vi "RLC Circuit.vi"() -> ()   [LabVIEW 2017]
uses:
  <vilib>/addons/_JKI.lib/REST Client/classes/REST Client/HTTP Header.ctl
  <vilib>/addons/_JKI.lib/REST Client/classes/REST Client/REST Client.lvclass
  <vilib>/httpClient/MultipartData.ctl
  <vilib>/LVH/i3 JSON/JSON Parsing/Get Object Parameter Files/Get Object Parameter - Object.vi
  <vilib>/LVH/i3 JSON/JSON Generation/Create Value Files/Create Value - String.vi
  <vilib>/LVH/i3 JSON/JSON Generation/Add Object Parameter Files/Add Object Parameter - Object.vi
  <vilib>/Analysis/NI_AALBase.lvlib
  <vilib>/httpClient/LabVIEWHTTPClient.lvlib
  <vilib>/LVH/i3 JSON/i3-json.lvlib
panel:
  out "error out  2":errorcluster
  out "Local Cluster":T2={"Base URL Getting"="https://api.dev.enlil.io/api", "Path"="/v1/document_revisions/external/ALI00017/draft", "Default Headers ([JSON])"=[{"header"="Content-Type", "value"="application/json"}, {"header"="Authorization", "value"="apitoken 2096a662-4947-42f5-97bc-84cfdf20fe4e:bc240510-8f48-43e3-889a-471659905c2e"}]}
  out "error out 4":errorcluster={"status"=TRUE, "code"=0, "source"="Input has UNKNOWN type, Expecting JSON Object"}
  out "headers":string="HTTP/1.1 201 Created\r\nDate: Wed, 04 Mar 2020 22:35:49 GMT\r\nContent-Type: application/json; charset=utf-8\r\nContent-Length: 655\r\nConnection: keep-alive\r\nSet-Cookie: AWSALB=VxqNwSYeQG0m47IXiOZ1OzDZLcK+M/95m4sL+aiBIfyiuOveEpJhbIw2+MdgPGt87DC4Ig6JZd2B6jRkdLsrHcqbrtdnjQCVFvEQhCU/fEw1chZBYJ72zQdVEr3j; Expires=Wed, 11 Mar 2020 22:35:48 GMT; Path=/\r\nSet-Cookie: AWSALBCORS=VxqNwSYeQG0m47IXiOZ1OzDZLcK+M/95m4sL+aiBIfyiuOveEpJhbIw2+MdgPGt87DC4Ig6JZd2B6jRkdLsrHcqbrtdnjQCVFvEQhCU/fEw1chZBYJ72zQdVEr3j; Expires=Wed, 11 Mar 2020 22:35:48 GMT; Path=/; SameSite=None; Secure\r\nX-Powered-By: Express\r\nAccess-Control-Allow-Origin: *\r\nStrict-Transport-Security: max-age=15552000; includeSubDomains\r\nETag: W/\"28f-tuCZSSTEEmLl4gD3j85fY8Z3L9M\"\r\nVary: Accept-Encoding\r\n\r\n"
  out "error out 3":errorcluster
  in  "Tab Control":enum32{"Page 1", "Page 2"}(tab)
  in  "Start Sending":bool
  in  "Default Headers ([JSON])":T1[](array[typedef])=[{"header"="Content-Type", "value"="application/json"}, {"header"="Authorization", "value"="apitoken 2096a662-4947-42f5-97bc-84cfdf20fe4e:bc240510-8f48-43e3-889a-471659905c2e"}]
  in  "Base URL Getting":string="https://api.dev.enlil.io/api"
  in  "Path":string="/v1/document_revisions/external/ALI00017/draft"
  in  "Start Getting":bool
  out "Status Code":u16=200
  out "Status String":string="OK\r"
  in  "input cluster":T3={"Parameter Name Vin"="vin-k7ad0tyd", "Parameter Name R"="r-k7ad0z99", "Parameter Name L"="l-k7ad13xp", "Parameter Name C"="c-k7ad19ix"}
  in  "Parameter Name All":string="formInput"
  out "Vin":dbl
  out "R":dbl
  out "L":dbl
  out "C":dbl
  out "Response body":string="{\"createdAt\":\"2020-03-02T11:12:30.271Z\",\"updatedAt\":\"2020-03-04T22:15:54.912Z\",\"id\":\"483b4210-fea0-4e5f-86e6-7e2e9ef14ab9\",\"version\":1,\"revision\":1,\"revisionStage\":1,\"description\":\"<p>Luka - RLC _ TEST</p>\",\"name\":\"Luka\",\"status\":\"DRAFT\",\"deprecatedAt\":null,\"releasedAt\":null,\"obsoletedAt\":null,\"retrain\":false,\"formInput\":{\"vin-k7ad0tyd\":\"25\",\"r-k7ad0z99\":\"50\",\"l-k7ad13xp\":\"30\",\"c-k7ad19ix\":\"15\"},\"revisionChangeType\":\"NEXT_REVISION\",\"externalId\":null,\"renderHTML\":null,\"owner\":{\"createdAt\":\"2020-02-19T17:50:40.752Z\",\"updatedAt\":\"2020-02-19T17:50:40.752Z\",\"id\":\"796961dc-c686-4253-97f2-59d9360d9127\",\"active\":true,\"slackUserId\":null,\"user\":{\"createdAt\":\"2020-02-19T17:50:40.752Z\",\"updatedAt\":\"2020-02-19T17:50:40.752Z\",\"id\":\"70b289fa-7831-4846-97f9-a0727380590c\",\"email\":\"luka.stosic+labview@codecons.com\",\"name\":\"Company Admin\",\"permissions\":null,\"avatar\":null}},\"document\":{\"createdAt\":\"2020-03-02T11:12:30.271Z\",\"updatedAt\":\"2020-03-02T11:12:30.271Z\",\"id\":\"7317e6be-3b89-4428-84bb-8531eddc6023\",\"docId\":\"ALI00017\",\"documentType\":{\"createdAt\":\"2020-03-02T09:53:29.165Z\",\"updatedAt\":\"2020-03-02T09:53:29.165Z\",\"id\":\"f5ab57be-8a87-4427-8a37-ad589c6c9a93\",\"documentTypeName\":\"Ali Document\",\"documentTypeAcronym\":\"ALI\",\"group\":\"OTHER\",\"privateNumberPool\":false,\"isQms\":true,\"startingNumber\":1,\"pageDetails\":null},\"referencedBy\":[],\"securityEmployees\":[],\"securityGroups\":[{\"createdAt\":\"2020-02-19T17:50:40.752Z\",\"updatedAt\":\"2020-03-02T11:11:52.054Z\",\"id\":\"e9b1c157-b17b-42e6-940a-b3ff64f3c84a\",\"name\":\"Everyone\",\"permissions\":[\"EMPLOYEE_GET\"],\"defaultForNewUsers\":true,\"tags\":[\"QMS_DEFAULT\",\"OWNERSHIP_CHANGE\"],\"isOfficial\":true,\"employees\":[{\"createdAt\":\"2020-02-19T18:14:19.813Z\",\"updatedAt\":\"2020-02-19T18:14:19.813Z\",\"id\":\"14618d18-3c6c-4a3d-854c-2505bd3d66b8\",\"active\":true,\"slackUserId\":null,\"user\":{\"createdAt\":\"2019-12-17T16:55:55.030Z\",\"updatedAt\":\"2019-12-17T16:55:58.645Z\",\"id\":\"ccba97cc-6396-4955-b83a-8af76ff01aa4\",\"email\":\"adarkazanli@shifamed.com\",\"name\":\"Ammar Darkazanli - Admin\",\"permissions\":null,\"avatar\":null}},{\"createdAt\":\"2020-02-19T17:50:40.752Z\",\"updatedAt\":\"2020-02-19T17:50:40.752Z\",\"id\":\"796961dc-c686-4253-97f2-59d9360d9127\",\"active\":true,\"slackUserId\":null,\"user\":{\"createdAt\":\"2020-02-19T17:50:40.752Z\",\"updatedAt\":\"2020-02-19T17:50:40.752Z\",\"id\":\"70b289fa-7831-4846-97f9-a0727380590c\",\"email\":\"luka.stosic+labview@codecons.com\",\"name\":\"Company Admin\",\"permissions\":null,\"avatar\":null}}]}],\"canAccess\":true},\"referenceTo\":[],\"changeRequest\":null,\"trainingRecords\":[],\"pdf\":null,\"attachments\":[],\"formTemplate\":null,\"formDocument\":{\"createdAt\":\"2020-03-02T11:11:42.254Z\",\"updatedAt\":\"2020-03-02T11:11:52.054Z\",\"id\":\"59fcbba9-0bd2-42e5-afd8-1e80379511c7\",\"version\":1,\"revision\":1,\"revisionStage\":1,\"description\":\"<p><span style=\\\"color: rgb(77,77,77);background-color: rgb(255,255,255);font-size: 14px;font-family: Open Sans\\\", sans-serif;\\\">RLC circuit which imports the data from the api ( Vin - R - L - C ) and exports 2 images to the api. One for Series Circuit and another for Parallel Circuit.</span></p>\",\"name\":\"RLC - Luka Test\",\"status\":\"RELEASED\",\"deprecatedAt\":null,\"releasedAt\":\"2020-03-02T11:11:53.929Z\",\"obsoletedAt\":null,\"retrain\":false,\"formInput\":null,\"revisionChangeType\":\"NEXT_REVISION\",\"externalId\":null,\"renderHTML\":null,\"formTemplate\":{\"createdAt\":\"2020-03-02T11:11:42.254Z\",\"updatedAt\":\"2020-03-02T11:11:42.254Z\",\"id\":\"64323185-9de3-4394-af92-7432be18ca58\",\"schema\":[{\"type\":\"textfield\",\"index\":0,\"name\":\"vin-k7ad0tyd\",\"label\":\"Vin\",\"rules\":\"\",\"applicableOn\":[\"ON_STATE_TO_IN_REVIEW\"],\"formValuesRules\":{}},{\"type\":\"textfield\",\"index\":1,\"name\":\"r-k7ad0z99\",\"label\":\"R\",\"rules\":\"\",\"applicableOn\":[\"ON_STATE_TO_IN_REVIEW\"],\"formValuesRules\":{}},{\"type\":\"textfield\",\"index\":2,\"name\":\"l-k7ad13xp\",\"label\":\"L\",\"rules\":\"\",\"applicableOn\":[\"ON_STATE_TO_IN_REVIEW\"],\"formValuesRules\":{}},{\"type\":\"textfield\",\"index\":3,\"name\":\"c-k7ad19ix\",\"label\":\"C\",\"rules\":\"\",\"applicableOn\":[\"ON_STATE_TO_IN_REVIEW\"],\"formValuesRules\":{}}]},\"document\":{\"createdAt\":\"2020-03-02T11:11:42.254Z\",\"updatedAt\":\"2020-03-02T11:11:42.254Z\",\"id\":\"307b5404-5fb5-4901-b94d-3c29afee9a02\",\"docId\":\"FM00016\"}}}"
  out "error out":errorcluster
  in  "PUT Path":string="/v1/document_revisions/external/0b9ed9ad-4393-4a37-838e-578edaaebe9e"
  out "Response body Putting":string="{\"createdAt\":\"2020-02-22T11:56:35.610Z\",\"updatedAt\":\"2020-03-04T22:35:50.355Z\",\"id\":\"0b9ed9ad-4393-4a37-838e-578edaaebe9e\",\"version\":1,\"revision\":1,\"revisionStage\":1,\"description\":\"<p>Test Ali</p>\",\"name\":\"Test Ali\",\"status\":\"DRAFT\",\"deprecatedAt\":null,\"releasedAt\":null,\"obsoletedAt\":null,\"retrain\":false,\"formInput\":{\"r-1-k6tm7v7p\":\"300,000000\",\"r-2-k6tm82gj\":\"220,000000\",\"r-3-k6tm86pp\":\"700,000000\",\"r-4-k6tm8czn\":\"1200,000000\",\"vin-k6tm7pik\":\"110,000000\",\"vout-k6tm8iia\":\"-22,935223\"},\"revisionChangeType\":\"NEXT_REVISION\",\"externalId\":null,\"renderHTML\":null,\"owner\":{\"createdAt\":\"2020-02-19T17:50:40.752Z\",\"updatedAt\":\"2020-02-19T17:50:40.752Z\",\"id\":\"796961dc-c686-4253-97f2-59d9360d9127\",\"active\":true,\"slackUserId\":null,\"user\":{\"createdAt\":\"2020-02-19T17:50:40.752Z\",\"updatedAt\":\"2020-02-19T17:50:40.752Z\",\"id\":\"70b289fa-7831-4846-97f9-a0727380590c\",\"email\":\"luka.stosic+labview@codecons.com\",\"name\":\"Company Admin\",\"permissions\":null,\"avatar\":null}},\"document\":{\"createdAt\":\"2020-02-22T11:56:35.610Z\",\"updatedAt\":\"2020-02-22T11:56:35.610Z\",\"id\":\"575eb1d7-b8d2-41b8-9d9e-9423dadb7d63\",\"docId\":\"CP00004\",\"documentType\":{\"createdAt\":\"2020-02-19T17:50:40.752Z\",\"updatedAt\":\"2020-02-19T17:50:40.752Z\",\"id\":\"baa29555-e386-488c-b5c3-d6ee972e153c\",\"documentTypeName\":\"Clinical Protocol\",\"documentTypeAcronym\":\"CP\",\"group\":\"OTHER\",\"privateNumberPool\":false,\"isQms\":true,\"startingNumber\":1,\"pageDetails\":null},\"referencedBy\":[],\"securityEmployees\":[],\"securityGroups\":[],\"canAccess\":true},\"referenceTo\":[],\"changeRequest\":null,\"trainingRecords\":[],\"pdf\":null,\"attachments\":[],\"formTemplate\":null,\"formDocument\":{\"createdAt\":\"2020-02-20T20:27:52.637Z\",\"updatedAt\":\"2020-02-24T13:01:24.572Z\",\"id\":\"75c93c40-92be-411d-bc74-84a119fc04b8\",\"version\":2,\"revision\":2,\"revisionStage\":1,\"description\":\"<p>test</p>\",\"name\":\"Form Notebook\",\"status\":\"DEPRECATED\",\"deprecatedAt\":\"2020-02-24T13:01:25.722Z\",\"releasedAt\":\"2020-02-20T20:28:22.146Z\",\"obsoletedAt\":null,\"retrain\":false,\"formInput\":null,\"revisionChangeType\":\"NEXT_REVISION\",\"externalId\":null,\"renderHTML\":null,\"formTemplate\":{\"createdAt\":\"2020-02-20T20:27:52.637Z\",\"updatedAt\":\"2020-02-20T20:27:52.637Z\",\"id\":\"9a42de21-a365-4d40-b1db-612758cdd974\",\"schema\":[{\"type\":\"textfield\",\"index\":0,\"name\":\"vin-k6tm7pik\",\"label\":\"Vin\",\"rules\":\"\",\"applicableOn\":[\"ON_STATE_TO_IN_REVIEW\"],\"formValuesRules\":{}},{\"type\":\"textfield\",\"index\":1,\"name\":\"r-1-k6tm7v7p\",\"label\":\"R1\",\"rules\":\"\",\"applicableOn\":[\"ON_STATE_TO_IN_REVIEW\"],\"formValuesRules\":{}},{\"type\":\"textfield\",\"index\":2,\"name\":\"r-2-k6tm82gj\",\"label\":\"R2\",\"rules\":\"\",\"applicableOn\":[\"ON_STATE_TO_IN_REVIEW\"],\"formValuesRules\":{}},{\"type\":\"textfield\",\"index\":3,\"name\":\"r-3-k6tm86pp\",\"label\":\"R3\",\"rules\":\"\",\"applicableOn\":[\"ON_STATE_TO_IN_REVIEW\"],\"formValuesRules\":{}},{\"type\":\"textfield\",\"index\":4,\"name\":\"r-4-k6tm8czn\",\"placeholder\":\"\",\"label\":\"R4\",\"rules\":\"\",\"applicableOn\":[\"ON_STATE_TO_IN_REVIEW\"],\"formValuesRules\":{}},{\"type\":\"textfield\",\"index\":5,\"name\":\"vout-k6tm8iia\",\"label\":\"Vout\",\"rules\":\"\",\"applicableOn\":[\"ON_STATE_TO_IN_REVIEW\"],\"formValuesRules\":{}},{\"type\":\"textfield\",\"index\":6,\"name\":\"initial-frequency-k6v75gp5\",\"label\":\"Initial Frequency\",\"rules\":\"\",\"applicableOn\":[\"ON_STATE_TO_IN_REVIEW\"],\"formValuesRules\":{}},{\"type\":\"textfield\",\"index\":7,\"name\":\"final-frequency-k6v7609o\",\"label\":\"Final Frequency\",\"rules\":\"\",\"applicableOn\":[\"ON_STATE_TO_IN_REVIEW\"],\"formValuesRules\":{}}]},\"document\":{\"createdAt\":\"2020-02-19T17:54:13.053Z\",\"updatedAt\":\"2020-02-19T17:54:13.053Z\",\"id\":\"316835f7-c3f4-4050-a09b-2d99776d6260\",\"docId\":\"FM00001\"}}}"
  out "Status String":string="OK\r"
  in  "Default Headers ([JSON]) PUT":T1[](array[typedef])=[{"header"="Content-Type", "value"="application/json"}, {"header"="Authorization", "value"="apitoken 2096a662-4947-42f5-97bc-84cfdf20fe4e:bc240510-8f48-43e3-889a-471659905c2e"}]
  in  "Base URL Posting":string="https://api.dev.enlil.io/api"
  in  "Same Params?":bool
  out "Status Code 2":u16=200
  out "body":string="{\"company\":{\"_addresses\":[],\"_acctCodes\":[],\"createdAt\":\"2020-02-19T17:50:40.752Z\",\"updatedAt\":\"2020-02-19T17:50:40.752Z\",\"id\":\"a64ce667-962d-4ce0-9671-2a28305a948e\",\"name\":\"LabView\",\"slackIntegrationEnabled\":true,\"teamId\":null,\"botToken\":null,\"maxRevisionStages\":3,\"numOfDocDigits\":5,\"whiteLabeling\":null,\"remoteValidatorBundleName\":null},\"name\":\"Series\",\"type\":\"png\",\"s3link\":\"a64ce667-962d-4ce0-9671-2a28305a948e/2020-03-04T22:35:49.127Z_Series.png\",\"importMetadataJson\":{},\"cleanCopyStatus\":\"NOT_REQUIRED\",\"s3linkCleanCopy\":null,\"createdAt\":\"2020-03-04T22:35:49.127Z\",\"updatedAt\":\"2020-03-04T22:35:49.127Z\",\"id\":\"7de0ce76-9aaf-4a44-b9a1-fc2d4d2266e7\"}"
  out "ID":string="7de0ce76-9aaf-4a44-b9a1-fc2d4d2266e7"
  in  "Upload Authorization":cluster{"header":string, "value":string}={"header"="Authorization", "value"="apitoken 475eef11-95b9-4f32-9221-3162004815ef:f20a91a0-c04e-4d32-b0b4-337e6e91bde7"}
  in  "Upload url":string="https://api.dev.enlil.io/api/v1/attachments/external/upload"
  out "String":string="ERROR_CREATING_JSON"
  in  "Start Plotting":bool=TRUE
  in  "Vinput frequency":dbl(slide)=651.0204081632653 scale=50.0..1000.0
  in  "Parallel:TRUE\nSeries:FALSE":bool
  in  "Impedence (H)":dbl=0.01
  in  "Capacitave (F)":dbl=7.5e-06
  in  "Resistence (R)":dbl=10.0
  in  "Vin amplitude":dbl=240.0 format="%0.2f"
  out "Vinput":dbl[](graph)=[233.84881554845646, 179.45505549600446, -25.96921427714383, -209.53762906479267, -216.75784995042574, -41.55329337025555, 168.62277772616747, 236.88485258479605, 105.78313726153381, -114.34633543694304, -238.24120901539771, -161.63077426122916, 51.00914239165065, 220.71944218561416, 204.6708634324726, 16.369991514676656, -185.70796879866788, -231.49292800738712, -82.45197486133672, 135.9810818192522, 239.97159998927566, 142.00050183871045, -75.47911678246386, -229.435033330003, -190.29697469904485, 8.996221426702972, 200.7181407006107, 223.51440326106132, 58.19953035572229, -156.0964353966462, -239.02065384235954, -120.78357825926923, 99.10572071742891, 235.58701831555533, 173.79679126133473, -34.261914546322984, -213.48557637251054, -213.03842687244614, -33.296789893575706, 174.46763605481402, 235.39899602867686, 98.21707209595816, -121.62496091495767, -239.10665756763365, -155.35467891243366, 59.144780100903446, 223.86761810318018, 200.18205279446192, 8.022005744805721, -190.8894120771005, -229.14709335986316, -74.5531315640869, 142.78521728885485, 239.95462418514296, 135.17670170504283, -83.366787894012, -231.74826152425555, -185.08893249693114, 17.342412768146225, 205.17827376039116, 220.33480184680573, 50.05616712795717, -162.3500544405009, -238.12144336202775, -113.48831948237336, 106.65729186320311, 237.03945179199007, 167.9277098682314, -42.513054787873806, -217.17456364835783, -209.06058615929993, -24.99989709461981, 180.1008634840137, 233.62759825458804, 90.53186868901375, -128.7560541600924, -239.68206747335293, -148.89013686265477, 67.20867463028469, 226.7442404736595, 195.45041942513296, -0.3357107941088627, -195.83930468579715, -226.5233011116992, -66.56385461007552, 149.41615293362366, 239.64658114292064, 128.1889309484015, -91.15333430018511, -233.78037687611342, -179.65637566175587, 25.667567598066995, 209.38952362549625, 216.88793222522588, 41.85208529394629, -168.40674132623874, -236.9333893093429, -106.05539829614163, 114.07948670108303, 238.204354161992, 161.85493056809338, -50.712626290064065, -220.60011611595087, -204.82915296955153, -16.67267918293669, 185.5156268551391, 231.57280798492926, 82.73684926559056, -135.7309650887793, -239.96674075473075, -142.24498966269664, 75.19104439888136, 229.34581992699668, 190.48170284072964, -8.69302011275931, -200.55164235776843, -223.6247339478602, -58.49383506831439, 155.86584536590743, 239.04784452162517, 121.04566580095585, -98.82931084597281, -235.52891441053583, -174.00589393661213, 33.961587424832324, 213.34678200961326, 213.17797548192996, 33.59723648308025]
  in  "Fo?":bool=TRUE
  out "Current - Frequency Response":cluster{"X":dbl[], "Y":dbl[]}[](graph)=[{"X"=[0.0, 1.0, 2.0, 3.0, 4.0, 5.0, 6.0, 7.0, 8.0, 9.0, 10.0, 11.0, 12.0, 13.0, 14.0, 15.0, 16.0, 17.0, 18.0, 19.0, 20.0, 21.0, 22.0, 23.0, 24.0, 25.0, 26.0, 27.0, 28.0, 29.0, 30.0, 31.0, 32.0, 33.0, 34.0, 35.0, 36.0, 37.0, 38.0, 39.0, 40.0, 41.0, 42.0, 43.0, 44.0, 45.0, 46.0, 47.0, 48.0, 49.0, 50.0, 51.0, 52.0, 53.0, 54.0, 55.0, 56.0, 57.0, 58.0, 59.0, 60.0, 61.0, 62.0, 63.0, 64.0, 65.0, 66.0, 67.0, 68.0, 69.0, 70.0, 71.0, 72.0, 73.0, 74.0, 75.0, 76.0, 77.0], "Y"=[0.0, 0.0001279093439907941, 0.0005116286274565821, 0.0011511316053372826, 0.002046374537398417, 0.003197296190529561, 0.004603817841962096, 0.006265843283406199, 0.008183258826106956, 0.010355933306819496, 0.012783718094703, 0.01546644709913344, 0.018403936778434823, 0.0215959861495288, 0.025042376798502308, 0.028742872892093246, 0.0326972211900935, 0.036905151058669455, 0.04136637448459942, 0.04608058609042774, 0.05104746315053532, 0.05626666560812573, 0.061737836093127274, 0.06746059994101006, 0.07343456521251747, 0.07965932271431238, 0.08613444602053646, 0.09285949149528333, 0.09983399831598429, 0.10705748849770579, 0.11452946691835893, 0.12224942134482022, 0.13021682245996197, 0.13843112389059317, 0.14689176223630918, 0.1555981570992499, 0.164549711114766, 0.17374580998299163, 0.18318582250132406, 0.19286910059780862, 0.2027949793654282, 0.21296277709729705, 0.22337179532275803, 0.2340213188443811, 0.24491061577586495, 0.2560389375808376, 0.2674055191125576, 0.279009578654514, 0.2908503179619234, 0.3029269223041252, 0.3152385605078709, 0.3277843850015102, 0.3405635318600694, 0.35357512085122345, 0.36681825548215957, 0.38029202304733173, 0.39399549467710293, 0.40792772538727934, 0.4220877541295284, 0.43647460384268355, 0.4510872815049364, 0.46592477818690975, 0.48098606910561315, 0.49627011367928237, 0.5117758555830951, 0.5275022228057681, 0.5434481277070307, 0.5596124670759731, 0.5759941221902721, 0.5925919588762874, 0.6094048275700303, 0.6264315633790047, 0.6436709861449139, 0.6611219005072388, 0.6787830959676776, 0.6966533469554558, 0.7147314128934922, 0.7330160382654349]}, {"X"=[581.1516831325472, 581.1516831325472, 581.1516831325472, 581.1516831325472, 581.1516831325472, 581.1516831325472, 581.1516831325472, 581.1516831325472, 581.1516831325472, 581.1516831325472, 581.1516831325472, 581.1516831325472, 581.1516831325472, 581.1516831325472, 581.1516831325472, 581.1516831325472, 581.1516831325472, 581.1516831325472, 581.1516831325472, 581.1516831325472, 581.1516831325472, 581.1516831325472, 581.1516831325472, 581.1516831325472, 581.1516831325472, 581.1516831325472, 581.1516831325472, 581.1516831325472, 581.1516831325472, 581.1516831325472, 581.1516831325472, 581.1516831325472, 581.1516831325472, 581.1516831325472, 581.1516831325472, 581.1516831325472, 581.1516831325472, 581.1516831325472, 581.1516831325472, 581.1516831325472, 581.1516831325472, 581.1516831325472, 581.1516831325472, 581.1516831325472, 581.1516831325472, 581.1516831325472, 581.1516831325472, 581.1516831325472, 581.1516831325472, 581.1516831325472, 581.1516831325472, 581.1516831325472, 581.1516831325472, 581.1516831325472, 581.1516831325472, 581.1516831325472, 581.1516831325472, 581.1516831325472, 581.1516831325472, 581.1516831325472, 581.1516831325472, 581.1516831325472, 581.1516831325472, 581.1516831325472, 581.1516831325472, 581.1516831325472, 581.1516831325472, 581.1516831325472, 581.1516831325472, 581.1516831325472, 581.1516831325472, 581.1516831325472, 581.1516831325472, 581.1516831325472, 581.1516831325472, 581.1516831325472, 581.1516831325472, 581.1516831325472], "Y"=[0.0, 0.0, 0.0, 0.0, 0.0, 0.0, 0.0, 0.0, 0.0, 0.0, 0.0, 0.0, 0.0, 0.0, 0.0, 0.0, 0.0, 0.0, 0.0, 0.0, 0.0, 0.0, 0.0, 0.0, 0.0, 0.0, 0.0, 0.0, 0.0, 0.0, 0.0, 0.0, 0.0, 0.0, 0.0, 0.0, 0.0, 0.0, 0.0, 0.0, 0.0, 0.0, 0.0, 0.0, 0.0, 0.0, 0.0, 0.0, 0.0, 0.0, 0.0, 0.0, 0.0, 0.0, 0.0, 0.0, 0.0, 0.0, 0.0, 0.0, 0.0, 0.0, 0.0, 0.0, 0.0, 0.0, 0.0, 0.0, 0.0, 0.0, 0.0, 0.0, 0.0, 0.0, 0.0, 0.0, 0.0, 0.0]}, {"X"=[290.5758415662736, 290.5758415662736, 290.5758415662736, 290.5758415662736, 290.5758415662736, 290.5758415662736, 290.5758415662736, 290.5758415662736, 290.5758415662736, 290.5758415662736, 290.5758415662736, 290.5758415662736, 290.5758415662736, 290.5758415662736, 290.5758415662736, 290.5758415662736, 290.5758415662736, 290.5758415662736, 290.5758415662736, 290.5758415662736, 290.5758415662736, 290.5758415662736, 290.5758415662736, 290.5758415662736, 290.5758415662736, 290.5758415662736, 290.5758415662736, 290.5758415662736, 290.5758415662736, 290.5758415662736, 290.5758415662736, 290.5758415662736, 290.5758415662736, 290.5758415662736, 290.5758415662736, 290.5758415662736, 290.5758415662736, 290.5758415662736, 290.5758415662736, 290.5758415662736, 290.5758415662736, 290.5758415662736, 290.5758415662736, 290.5758415662736, 290.5758415662736, 290.5758415662736, 290.5758415662736, 290.5758415662736, 290.5758415662736, 290.5758415662736, 290.5758415662736, 290.5758415662736, 290.5758415662736, 290.5758415662736, 290.5758415662736, 290.5758415662736, 290.5758415662736, 290.5758415662736, 290.5758415662736, 290.5758415662736, 290.5758415662736, 290.5758415662736, 290.5758415662736, 290.5758415662736, 290.5758415662736, 290.5758415662736, 290.5758415662736, 290.5758415662736, 290.5758415662736, 290.5758415662736, 290.5758415662736, 290.5758415662736, 290.5758415662736, 290.5758415662736, 290.5758415662736, 290.5758415662736, 290.5758415662736, 290.5758415662736], "Y"=[0.0, 0.0, 0.0, 0.0, 0.0, 0.0, 0.0, 0.0, 0.0, 0.0, 0.0, 0.0, 0.0, 0.0, 0.0, 0.0, 0.0, 0.0, 0.0, 0.0, 0.0, 0.0, 0.0, 0.0, 0.0, 0.0, 0.0, 0.0, 0.0, 0.0, 0.0, 0.0, 0.0, 0.0, 0.0, 0.0, 0.0, 0.0, 0.0, 0.0, 0.0, 0.0, 0.0, 0.0, 0.0, 0.0, 0.0, 0.0, 0.0, 0.0, 0.0, 0.0, 0.0, 0.0, 0.0, 0.0, 0.0, 0.0, 0.0, 0.0, 0.0, 0.0, 0.0, 0.0, 0.0, 0.0, 0.0, 0.0, 0.0, 0.0, 0.0, 0.0, 0.0, 0.0, 0.0, 0.0, 0.0, 0.0]}, {"X"=[871.7275246988208, 871.7275246988208, 871.7275246988208, 871.7275246988208, 871.7275246988208, 871.7275246988208, 871.7275246988208, 871.7275246988208, 871.7275246988208, 871.7275246988208, 871.7275246988208, 871.7275246988208, 871.7275246988208, 871.7275246988208, 871.7275246988208, 871.7275246988208, 871.7275246988208, 871.7275246988208, 871.7275246988208, 871.7275246988208, 871.7275246988208, 871.7275246988208, 871.7275246988208, 871.7275246988208, 871.7275246988208, 871.7275246988208, 871.7275246988208, 871.7275246988208, 871.7275246988208, 871.7275246988208, 871.7275246988208, 871.7275246988208, 871.7275246988208, 871.7275246988208, 871.7275246988208, 871.7275246988208, 871.7275246988208, 871.7275246988208, 871.7275246988208, 871.7275246988208, 871.7275246988208, 871.7275246988208, 871.7275246988208, 871.7275246988208, 871.7275246988208, 871.7275246988208, 871.7275246988208, 871.7275246988208, 871.7275246988208, 871.7275246988208, 871.7275246988208, 871.7275246988208, 871.7275246988208, 871.7275246988208, 871.7275246988208, 871.7275246988208, 871.7275246988208, 871.7275246988208, 871.7275246988208, 871.7275246988208, 871.7275246988208, 871.7275246988208, 871.7275246988208, 871.7275246988208, 871.7275246988208, 871.7275246988208, 871.7275246988208, 871.7275246988208, 871.7275246988208, 871.7275246988208, 871.7275246988208, 871.7275246988208, 871.7275246988208, 871.7275246988208, 871.7275246988208, 871.7275246988208, 871.7275246988208, 871.7275246988208], "Y"=[0.0, 0.0, 0.0, 0.0, 0.0, 0.0, 0.0, 0.0, 0.0, 0.0, 0.0, 0.0, 0.0, 0.0, 0.0, 0.0, 0.0, 0.0, 0.0, 0.0, 0.0, 0.0, 0.0, 0.0, 0.0, 0.0, 0.0, 0.0, 0.0, 0.0, 0.0, 0.0, 0.0, 0.0, 0.0, 0.0, 0.0, 0.0, 0.0, 0.0, 0.0, 0.0, 0.0, 0.0, 0.0, 0.0, 0.0, 0.0, 0.0, 0.0, 0.0, 0.0, 0.0, 0.0, 0.0, 0.0, 0.0, 0.0, 0.0, 0.0, 0.0, 0.0, 0.0, 0.0, 0.0, 0.0, 0.0, 0.0, 0.0, 0.0, 0.0, 0.0, 0.0, 0.0, 0.0, 0.0, 0.0, 0.0]}] caption="XY Graph"
  out "Frequency (H)":dbl(slide)=77.0 scale=0.0..3000.0
  out "XL":dbl=4.838052686528282
  out "Xc":dbl=275.59297505090103
  out "Supply Current (A)":dbl(slide)=0.7330160382654349 scale=0.0..100.0
  in  "Reset":bool
  out "Fo":dbl=581.1516831325472
  out "Ifo":dbl=23.998638408079707
  out "Building Pic":picture
  out "Fl":dbl=290.5758415662736
  out "Fh":dbl=871.7275246988208
  out "Half Band":dbl=290.5758415662736
  in  "stop":bool
  out "Final Pic Parallel Circuit":picture
  out "Final Pic Series Circuit":picture
  out "Case":string="Parallel"
  in  "Toggle":bool=TRUE
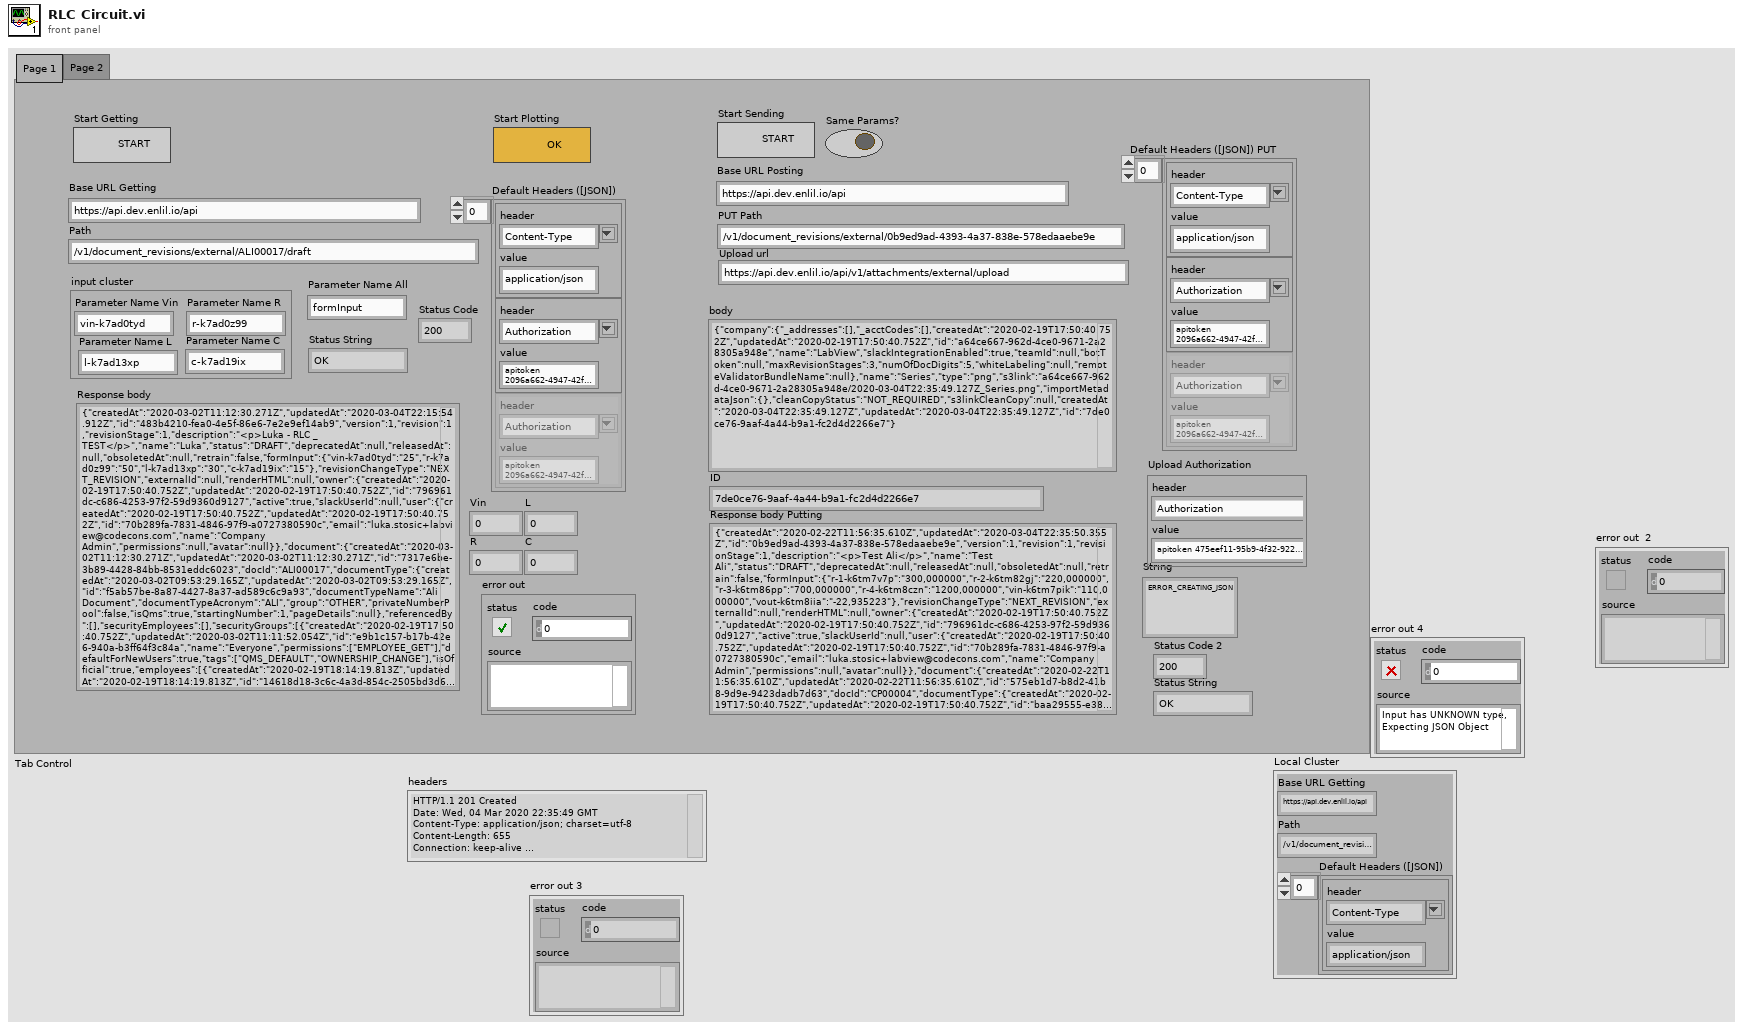
[diagram p1: front panel]
types:
  T1 = typedef "REST Client.lvlib/REST Client.lvclass/HTTP Header.ctl" = cluster{"header":string, "value":string}
  T2 = cluster{"Base URL Getting":string, "Path":string, "Default Headers ([JSON])":T1[]}
  T3 = cluster{"Parameter Name Vin":string, "Parameter Name R":string, "Parameter Name L":string, "Parameter Name C":string}
  T4 = typedef "LabVIEWHTTPClient.lvlib/MultipartData.ctl" = cluster{"Name":string, "Value":string, "File":path, "Filename":string, "MIME type":string}
  T5 = cluster{"Vinput":dbl, "R1":dbl, "R2":dbl, "R3":dbl, "R4":dbl}
  T6 = typedef "LabVIEWHTTPClient.lvlib/ClientHandle.ctl" = refnum<k1>
  T7 = typedef "imagedata.ctl" = cluster{"image type":i32, "image depth":i32, "image":u8[], "mask":u8[], "colors":u32[], "Rectangle":cluster{"left":i16, "top":i16, "right":i16, "bottom":i16}}
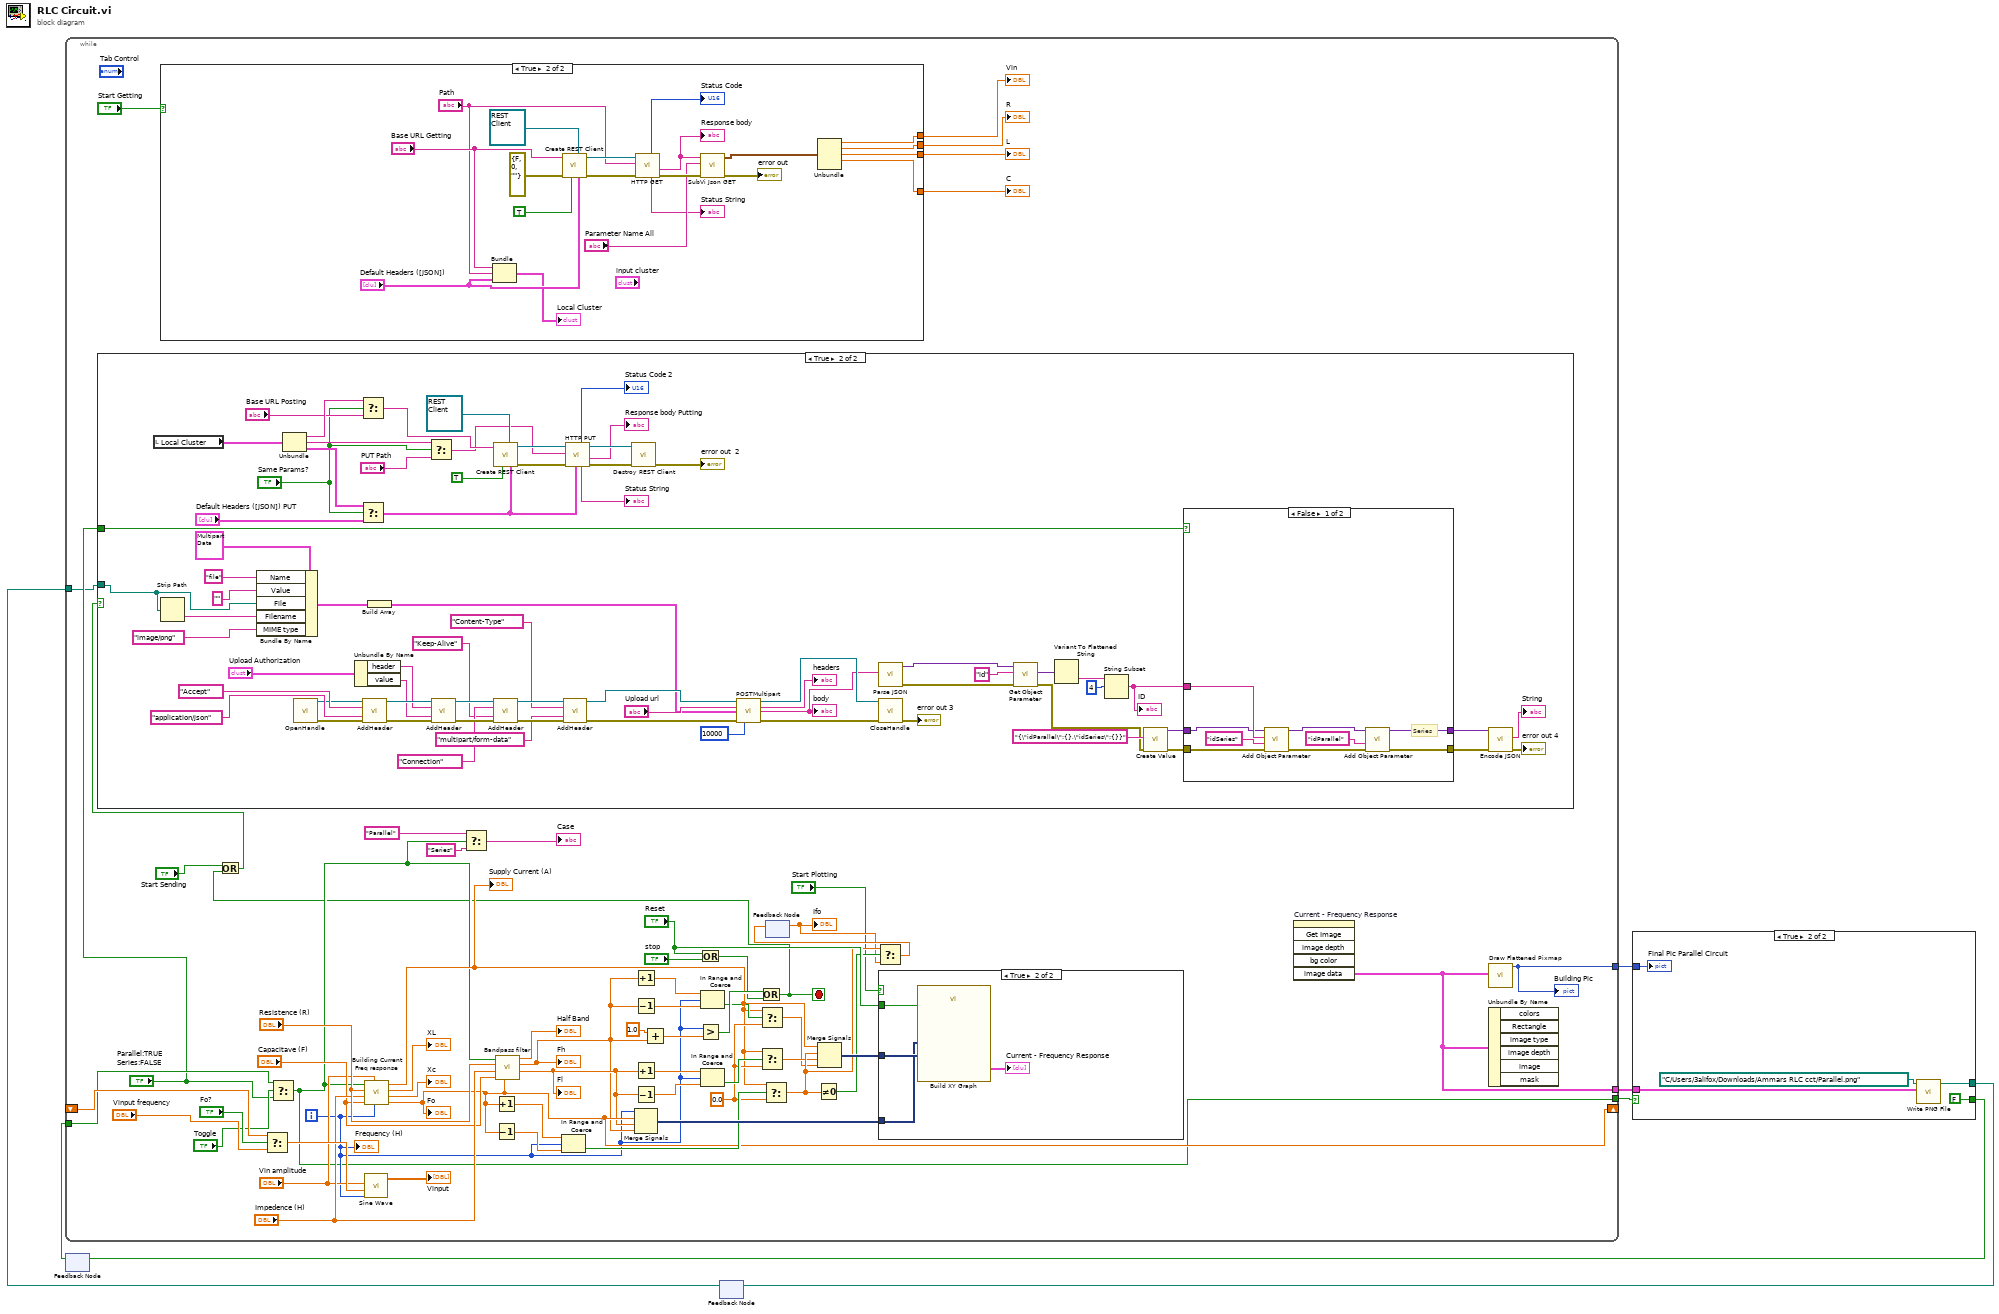
[diagram p0: block diagram]
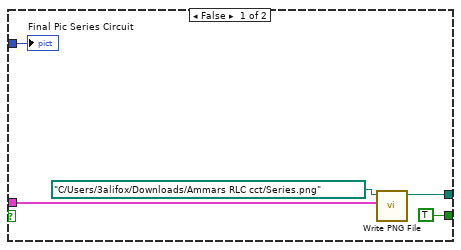
[diagram p2: hidden frame]
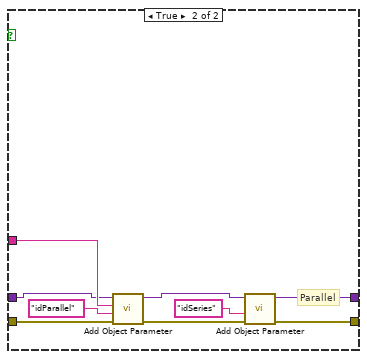
[diagram p4: hidden frame]
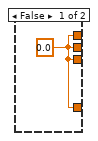
[diagram p6: hidden frame]
diagram:
  n1 = feedback #1() -> (w5:bool)  [unwired: 1 in]
  n2 = feedback #2() -> (w1:path)  [unwired: 1 in]
  n3 = while {
    tunnel: [w57] -> w7
    tunnel: [w20] -> w3
    tunnel: w5 -> [w21]
    shift-right: [w28] -> _
    shift-left: _ -> [w35]
    tunnel: [w14] -> w4
    tunnel: w1 -> [w11]
    i -> [w23]
    stop <- w10 stop-if-true
    w37 = 0.0 ("f")
    n4 = case shown="True" "Start Getting" {
      tunnel: [w161 w169] -> w18
      tunnel: [w161 w168] -> w17
      tunnel: [w161 w167] -> w16
      tunnel: [w161 w166] -> w15
      frame False {
        w161 = 0.0
      }
      frame True {
        n5 = Bundle("Base URL Getting"="Base URL Getting", "Path"="Path", "Default Headers ([JSON])"="Default Headers ([JSON])") -> (→"Local Cluster":T2)  [unwired: 1 in]
        n6 = call <vilib>:"Create REST Client.vi"("Default Headers ([JSON])"="Default Headers ([JSON])", "REST Client in"=refnum<class "REST Client.lvclass"> refnum, "Verify Server(true)"=TRUE, "error in (no error)"=errorcluster {"status"=FALSE, "code"=0, "source"=""}, "Base URL"="Base URL Getting") -> ("error out"=w170:errorcluster, "REST Client out"=w171:refnum<class "REST Client.lvclass">)  [unwired: 5 in]
        n7 = call-dynamic "HTTP GET.vi"("error in (no error)"=w170, "Path"="Path", "REST Client in"=w171) -> ("error out"=w176:errorcluster, "Response body"=w174:string, "Status String"=→"Status String":string, "Status Code"=→"Status Code":u16)  [unwired: 3 in, 2 out]
        "Response body" <- w174
        n8 = call "SubVi Json GET.vi"("error in (no error)"=w176, "Parameter Name All"="Parameter Name All", "Response Body"=w174) -> ("error out"=→"error out":errorcluster, "Cluster"=w177:T5)  [unwired: 7 in]
        n9 = Unbundle(w177) -> ("Vinput"=w166:dbl, "R1"=w168:dbl, "R2"=w167:dbl, "R3"=w169:dbl)  [unwired: 1 out]
      }
    }
    "C" <- w18
    "R" <- w17
    "L" <- w16
    "Vin" <- w15
    n10 = Select(t=w35, s="Fo?", f="Vinput frequency") -> (s? t:f=w66:dbl)
    n11 = Select(t=w21, s="Toggle", f="Parallel:TRUE\nSeries:FALSE") -> (s? t:f=w20:bool)
    n12 = call <vilib>:"Sine Wave.vi"("amplitude"="Vin amplitude", "frequency"=w66, "phase in"=w23) -> ("sine wave"=→"Vinput":dbl[])  [unwired: 2 in, 2 out]
    n13 = call "Building Current Freq response.vi"("F variable"=w23, "Vin"="Vin amplitude", "C"="Capacitave (F)", "L"="Impedence (H)", "R"="Resistence (R)", "Boolean"=w20) -> ("Fo"=w28:dbl, "Xc"=→"Xc":dbl, "Xl"=→"XL":dbl, "Supply Current"=w30:dbl)  [unwired: 2 in]
    "Supply Current (A)" <- w30
    "Fo" <- w28
    n14 = Select(t="Parallel", s=w20, f="Series") -> (s? t:f=→"Case":string)
    n15 = Increment(x=w28) -> (x+1=w45:dbl)
    n16 = Decrement(x=w28) -> (x-1=w53:dbl)
    n17 = call "Bandpass filter.vi"("Fr"=w28, "C"="Capacitave (F)", "L"="Impedence (H)", "R"="Resistence (R)", "Boolean"=w20) -> ("Fl"=w26:dbl, "Fh"=w25:dbl, "half"=→"Half Band":dbl)  [unwired: 4 in]
    "Fl" <- w26
    "Fh" <- w25
    n18 = In Range and Coerce(upper limit=w45, x=w23, lower limit=w53) -> (In Range?=w52:bool)  [unwired: 1 out]
    n19 = Increment(x=w25) -> (x+1=w40:dbl)
    n20 = Decrement(x=w25) -> (x-1=w39:dbl)
    n21 = Increment(x=w26) -> (x+1=w44:dbl)
    n22 = Decrement(x=w26) -> (x-1=w43:dbl)
    n23 = Merge Signals(w23, w28, w26, w25) -> (w62:dynamicdata)
    n24 = Add(x=1.0, y=w25) -> (x+y=w47:dbl)
    n25 = Or(x="Reset", y="stop") -> (x .or. y?=w59:bool)
    n26 = Greater?(x=w23, y=w47) -> (0:w61:bool)
    n27 = In Range and Coerce(upper limit=w40, x=w23, lower limit=w39) -> (In Range?=w38:bool)  [unwired: 1 out]
    n28 = In Range and Coerce(upper limit=w44, x=w23, lower limit=w43) -> (In Range?=w42:bool)  [unwired: 1 out]
    n29 = Or(x=w61, y=w59) -> (x .or. y?=w10:bool)
    n30 = Or(x="Start Sending", y=w10) -> (x .or. y?=w8:bool)
    n31 = case shown="True" w8 {
      tunnel: "Parallel:TRUE\nSeries:FALSE" -> [_ w78]
      tunnel: w11 -> [_ w69]
      frame False {
      }
      frame True {
        n32 = local read "Local Cluster"() -> (w135:T2)
        n33 = Strip Path(path=w69) -> (name=w110:string)  [unwired: 1 out]
        n34 = Bundle By Name(cluster=T4 {"Name"="", "Value"="", "File"=path "", "Filename"="", "MIME type"="application/octet-stream"} ("Element"), "Name"="file", "Value"="", "File"=w69, "Filename"=w110, "MIME type"="image/png") -> (w112:T4)
        n35 = Unbundle(w135) -> ("Base URL Getting"=w134:string, "Path"=w129:string, "Default Headers ([JSON])"=w131:T1[])
        n36 = call <vilib>:"OpenHandle.vi"() -> ("client handle out"=w122:T6, "error out"=w91:errorcluster)  [unwired: 14 in]
        n37 = Unbundle By Name("Upload Authorization") -> ("header"=w87:string, "value"=w86:string)
        n38 = Select(t=w134, s="Same Params?", f="Base URL Posting") -> (s? t:f=w132:string)
        n39 = Select(t=w131, s="Same Params?", f="Default Headers ([JSON]) PUT") -> (s? t:f=w120:T1[])
        n40 = call <vilib>:"AddHeader.vi"("client handle"=w122, "header"="Accept", "value"="application/json", "error in (no error)"=w91) -> ("client handle out"=w126:T6, "error out"=w125:errorcluster)  [unwired: 10 in]
        n41 = Build Array(w112) -> (w90:T4[])
        n42 = Select(t=w129, s="Same Params?", f="PUT Path") -> (s? t:f=w117:string)
        n43 = call <vilib>:"AddHeader.vi"("client handle"=w126, "header"=w87, "value"=w86, "error in (no error)"=w125) -> ("client handle out"=w100:T6, "error out"=w101:errorcluster)  [unwired: 10 in]
        n44 = call <vilib>:"Create REST Client.vi"("Default Headers ([JSON])"=w120, "REST Client in"=refnum<class "REST Client.lvclass"> refnum, "Verify Server(true)"=TRUE, "Base URL"=w132) -> ("error out"=w119:errorcluster, "REST Client out"=w121:refnum<class "REST Client.lvclass">)  [unwired: 6 in]
        n45 = call <vilib>:"AddHeader.vi"("client handle"=w100, "header"="Connection", "value"="Keep-Alive", "error in (no error)"=w101) -> ("client handle out"=w96:T6, "error out"=w97:errorcluster)  [unwired: 10 in]
        n46 = call <vilib>:"AddHeader.vi"("client handle"=w96, "header"="Content-Type", "value"="multipart/form-data", "error in (no error)"=w97) -> ("client handle out"=w95:T6, "error out"=w94:errorcluster)  [unwired: 10 in]
        n47 = call-dynamic "HTTP PUT.vi"("request specific headers"=w120, "error in (no error)"=w119, "Path"=w117, "REST Client in"=w121) -> ("error out"=w114:errorcluster, "Response body"=→"Response body Putting":string, "REST Client out"=w118:refnum<class "REST Client.lvclass">, "Status String"=→"Status String":string, "Status Code"=→"Status Code 2":u16)  [unwired: 2 in, 1 out]
        n48 = call-dynamic "Destroy REST Client.vi"("error in (no error)"=w114, "REST Client in"=w118) -> ("error out"=→"error out  2":errorcluster)  [unwired: 9 in]
        n49 = call <vilib>:"POSTMultipart.vi"("client handle"=w95, "url"="Upload url", "data"=w90, "error in (no error)"=w94, "timeout (10000)"=10000) -> ("client handle out"=w107:T6, "headers"=→"headers":string, "body"=w85:string, "error out"=w106:errorcluster)  [unwired: 7 in]
        "body" <- w85
        n50 = call <vilib>:"Parse JSON.vi"("JSON String"=w85) -> ("error out"=w84:errorcluster, "JSON Tree"=w83:variant)  [unwired: 7 in, 2 out]
        n51 = call <vilib>:"CloseHandle.vi"("client handle"=w107, "error in (no error)"=w106) -> ("error out"=→"error out 3":errorcluster)  [unwired: 13 in]
        n52 = call-poly <vilib>:"Get Object Parameter.vi"("error in (no error)"=w84, "Parameter Name"="id", "JSON Tree In (JSON Object)"=w83) -> ("error out"=w68:errorcluster, "JSON Object"=w81:variant)  [unwired: 5 in, 2 out]
        n53 = Variant To Flattened String(Variant=w81) -> (data string=w80:string)  [unwired: 1 out]
        n54 = String Subset(string=w80, offset (0)=4) -> (substring=w76:string)  [unwired: 1 in]
        "ID" <- w76
        n55 = call-poly <vilib>:"Create Value.vi"("error in (no error)"=w68, "String"="{\"idParallel\":{},\"idSeries\":{}}") -> ("error out"=w77:errorcluster, "JSON Tree"=w75:variant)  [unwired: 8 in]
        n56 = case shown="False" w78 {
          tunnel: w76 -> [w147 w156]
          tunnel: [w140 w150] -> w73
          tunnel: w77 -> [w146 w154]
          tunnel: w75 -> [w145 w153]
          tunnel: [w141 w151] -> w74
          frame False {
            # "Series"
            n57 = call-poly <vilib>:"Add Object Parameter.vi"("error in (no error)"=w146, "Name"="idSeries", "JSON Object"=w147, "JSON Tree in (JSON Object)"=w145) -> ("error out"=w142:errorcluster, "JSON Tree out (JSON Object)"=w143:variant)  [unwired: 6 in]
            n58 = call-poly <vilib>:"Add Object Parameter.vi"("error in (no error)"=w142, "Name"="idParallel", "JSON Tree in (JSON Object)"=w143) -> ("error out"=w140:errorcluster, "JSON Tree out (JSON Object)"=w141:variant)  [unwired: 7 in]
          }
          frame True {
            # "Parallel"
            n59 = call-poly <vilib>:"Add Object Parameter.vi"("error in (no error)"=w154, "Name"="idParallel", "JSON Object"=w156, "JSON Tree in (JSON Object)"=w153) -> ("error out"=w148:errorcluster, "JSON Tree out (JSON Object)"=w152:variant)  [unwired: 6 in]
            n60 = call-poly <vilib>:"Add Object Parameter.vi"("error in (no error)"=w148, "Name"="idSeries", "JSON Tree in (JSON Object)"=w152) -> ("error out"=w150:errorcluster, "JSON Tree out (JSON Object)"=w151:variant)  [unwired: 7 in]
          }
        }
        n61 = call <vilib>:"Encode JSON.vi"("error in (no error)"=w73, "JSON Tree"=w74) -> ("error out"=→"error out 4":errorcluster, "String"=→"String":string)  [unwired: 4 in]
      }
    }
    n62 = Select(t=w30, s=w38, f=w37) -> (s? t:f=w36:dbl)
    n63 = Select(t=w30, s=w42, f=w37) -> (s? t:f=w41:dbl)
    n64 = Select(t=w30, s=w52, f=w37) -> (s? t:f=w50:dbl)
    n65 = feedback #3() -> (w48:dbl)  [unwired: 1 in]
    "Ifo" <- w48
    n66 = Not Equal To 0?(x=w50) -> (x != 0?=w51:bool)
    n67 = Merge Signals(w30, w50, w41, w36) -> (w63:dynamicdata)
    n68 = Select(t=w50, s=w51, f=w48) -> (s? t:f=w49:dbl)
    n69 = feedback-in #3(w49) -> ()
    n70 = case shown="True" "Start Plotting" {
      tunnel: w63 -> [_ w159]
      tunnel: w62 -> [_ w158]
      tunnel: "Reset" -> [_ w157]
      frame False {
      }
      frame True {
        n71 = call "Build XY Graph"("Reset"=w157, "Y Input"=w159, "X Input"=w158) -> ("XY Graph"=→"Current - Frequency Response":cluster{"X":dbl[], "Y":dbl[]}[])  [unwired: 7 in, 1 out]
      }
    }
    n72 = invoke on="Current - Frequency Response" class="XYGraph (strict)" method="Get Image"() -> ("image data"=w14:T7)  [unwired: 6 in, 5 out]
    n73 = call <vilib>:"Draw Flattened Pixmap.vi"("image data"=w14) -> ("new picture"=w57:picture)  [unwired: 8 in]
    "Building Pic" <- w57
    n74 = Unbundle By Name(w14) -> ()  [unwired: 6 out]
    "Frequency (H)" <- w23
  }
  n75 = case shown="True" w3 {
    tunnel: w7 -> [w185 w191]
    tunnel: [TRUE FALSE] -> w6
    tunnel: w4 -> [w184 w189]
    tunnel: [w182 w188] -> w2
    frame False {
      n76 = call <vilib>:"Write PNG File.vi"("image data"=w184, "path to PNG file"=path "C:/Users/3alifox/Downloads/Ammars RLC cct/Series.png" ("path to PNG file 2")) -> ("path"=w182:path)  [unwired: 8 in, 1 out]
      "Final Pic Series Circuit" <- w185
    }
    frame True {
      n77 = call <vilib>:"Write PNG File.vi"("image data"=w189, "path to PNG file"=path "C:/Users/3alifox/Downloads/Ammars RLC cct/Parallel.png" ("path to PNG file 2")) -> ("path"=w188:path)  [unwired: 8 in, 1 out]
      "Final Pic Parallel Circuit" <- w191
    }
  }
  n78 = feedback-in #1(w6) -> ()
  n79 = feedback-in #2(w2) -> ()
